vi "AnalogDelay_Example.vi"() -> ()   [LabVIEW 2019]
uses:
  <vilib>/Rock Robotics/WPI/ThirdParty/JAS_Junk/TrajLib/VI/TimeInterpDouble_New.vi
  <vilib>/Rock Robotics/WPI/ThirdParty/JAS_Junk/TrajLib/VI/TimeInterpDouble_AddSample.vi
  <vilib>/Rock Robotics/WPI/ThirdParty/JAS_Junk/TrajLib/VI/TimeInterpDouble_GetSample.vi
  <vilib>/Rock Robotics/WPI/ThirdParty/JAS_Junk/TrajLib/VI/TimeInterpDouble_SetMaxTime.vi
  <vilib>/Rock Robotics/WPI/ThirdParty/JAS_Junk/TrajLib/VI/TimeInterpDouble_CleanUp.vi
  <vilib>/Rock Robotics/WPI/ThirdParty/JAS_Junk/TrajLib/MathUtil_Interpolate.vi
  <vilib>/Rock Robotics/WPI/ThirdParty/JAS_Junk/TrajLib/MathUtil_Clamp.vi
  <vilib>/gmath/interp.llb/Search Ordered Table.vi
  <vilib>/Rock Robotics/WPI/ThirdParty/JAS_Junk/TrajLib/Trajectory_Library.lvlib
panel:
  out "Delayed Value":dbl=2000.0 format="%12.4f"
  out "Input Sinusoid Value":dbl=2000.0 format="%12.4f"
  out "Waveform Chart":cluster{dbl, "Output":dbl}(graph)
  out "Value is present\nin buffer.":bool
  in  "Input Sinusoid\nPeriod (ms)":dbl=2000.0
  in  "Delay (ms)":dbl=500.0 step=50.0
  # "ANALOG DELAY EXAMPLE"
  # "If the delay time is increased by more \nthan 1 second during runtime then the \nbuffer needs to be filled bofore a new \nvalue can be provided"
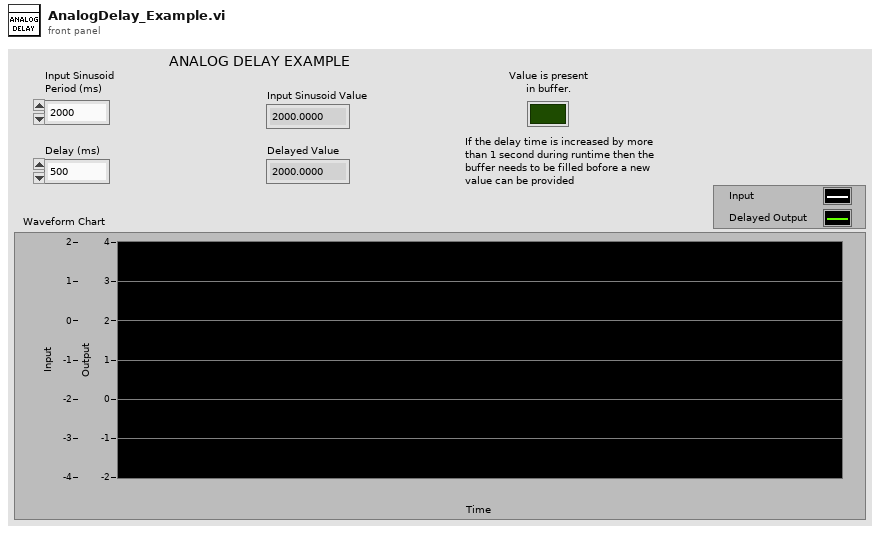
[diagram p1: front panel]
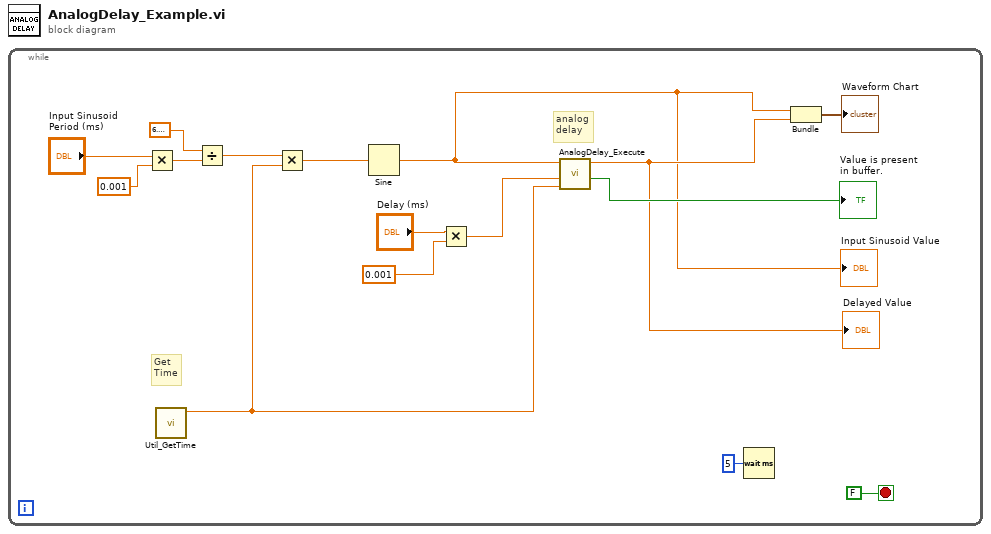
[diagram p0: block diagram]
diagram:
  n1 = while {
    stop <- FALSE stop-if-true
    # "analog\ndelay"
    # "Get\nTime"
    n2 = Multiply(x="Input Sinusoid\nPeriod (ms)", y=0.001) -> (x*y=w9:dbl)
    n3 = call <vilib>:"Util_GetTime.vi"() -> ("FPGA_Time_Seconds"=w4:dbl)  [unwired: 10 in, 1 out]
    n4 = Divide(x=6.283185307179586, y=w9) -> (x/y=w6:dbl)
    n5 = Multiply(x=w6, y=w4) -> (x*y=w5:dbl)
    n6 = Sine(x=w5) -> (sin(x)=w1:dbl)
    "Input Sinusoid Value" <- w1
    n7 = Multiply(x="Delay (ms)", y=0.001) -> (x*y=w11:dbl)
    n8 = call <vilib>:"AnalogDelay_Execute.vi"("Time"=w4, "Delay Time"=w11, "Input"=w1) -> ("IsPresent"=→"Value is present\nin buffer.":bool, "Output"=w2:dbl)  [unwired: 7 in]
    "Delayed Value" <- w2
    n9 = Wait (ms)(milliseconds to wait=u32 5) -> ()  [unwired: 1 out]
    n10 = Bundle(w1, "Output"=w2) -> (→"Waveform Chart":cluster{dbl, "Output":dbl})  [unwired: 1 in]
  }
